vi "Parse MAVLink Message Simple.vi"(8 "error in (no error)":errorcluster, 10 "Aircraft ID":u8, 11 "Mavlink Message":string) -> (0 "error in (no error) 2":errorcluster)   [LabVIEW 2014]
uses:
  Controls/MAVLink Command ACK.ctl
  Aircraft Information/Controls/Drone Information.ctl
  Aircraft Information/Controls/Base Mode.ctl
  Aircraft Information/Controls/Aircraft Mode.ctl
  Aircraft Information/Controls/Aircraft Extra Data.ctl
  Controls/MAVLink Optical Flow.ctl
  Controls/MAVLink EKF Status Report.ctl
  Aircraft Information/Controls/Aircraft Sensor Status Data.ctl
  GUI Design/Indicators/Sensor Status LED CLuster.ctl
  GUI Design/Indicators/Status LED.ctl
  Aircraft Information/Controls/Aircraft GPS Data.ctl
  Aircraft Information/Controls/GPS Fix Type.ctl
  Aircraft Information/Controls/Aircraft Attitude Data.ctl
  Controls/MAVLink Recieved Param.ctl
  Aircraft Information/Sub VI/Set Aircraft System Status.vi
  Aircraft Information/Sub VI/Set Aircraft Information.vi
  Aircraft Information/Sub VI/Set Aircraft Extra Data.vi
  Aircraft Information/Sub VI/Set Aircraft GPS.vi
  Aircraft Information/Sub VI/Set Aircraft Attitude.vi
panel:
  out "output cluster":T1
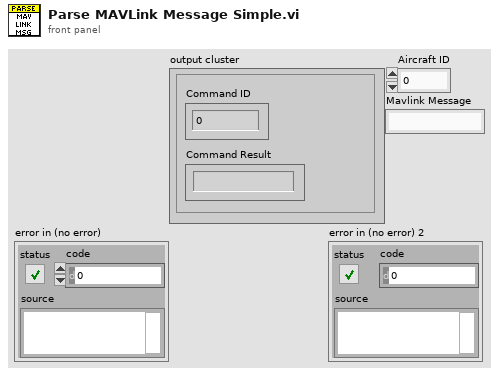
[diagram p1: front panel]
types:
  T1 = typedef "MAVLink Command ACK.ctl" = cluster{"Command ID":u16, "Command Result":string}
  T2 = typedef "Aircraft Attitude Data.ctl" = cluster{"Roll":sgl, "Pitch":sgl, "Yaw":sgl, "Timestamp":u32, "Update Frequency":dbl, "Altitude":sgl}
  T3 = typedef "Aircraft GPS Data.ctl" = cluster{"Latitude (degrees)":dbl, "Longitude (degrees)":dbl, "Altitude (m)":dbl, "Fix Type":T4, "HDOP (cm)":u16, "VDOP (cm)":u16, "Ground Speed (m/s)":dbl, "Coarse Over Ground (degrees)":u16, "Number of Satellites":u8}
  T4 = typedef "GPS Fix Type.ctl" = enum16{"No Fix 0", "No Fix 1", "2D Fix", "3D Fix", "DGPS", "RTK"}
  T5 = typedef "Aircraft Sensor Status Data.ctl" = cluster{"Sensor Status":T6, "CPU Load (%)":dbl, "Battery Voltage (V)":dbl, "Battery Current (A)":dbl, "Battery Remaining (%)":dbl, "Communication Drop Rate (%)":dbl, "Communication Errors (%)":dbl, "Status text":string}
  T6 = typedef "Sensor Status LED CLuster.ctl" = cluster{"3D Gyro":u32, "3D Accel":u32, "3D Mag":u32, "Abs. Pressure":u32, "Diff. Pressure":u32, "GPS":T7, "Optical Flow":u32, "Vision Position":u32, "Laser Position":u32, "External Ground Truth":u32, "Angular Rate Control":u32, "Attitude Stabilisation":u32, "Yaw Position":u32, "Z Altitude Control":u32, "XY Position Control":u32, "Motor Outputs":u32, "RC Receiver":u32, "3D Gyro 2":u32, "3D Accel 2":u32, "3D Mag 2":u32, "Geofence":u32, "AHRS":u32, "Terrain":u32}
  T7 = typedef "Status LED.ctl" = u32
  T8 = typedef "Aircraft Extra Data.ctl" = cluster{"Optical Flow":T9, "RNGFND Distance (m)":sgl, "RNGFND Voltage":sgl, "EKF Status Report":T10}
  T9 = typedef "MAVLink Optical Flow.ctl" = cluster{"Time (usec)":u64, "Flow Comp mx":sgl, "Flow Comp my":sgl, "Ground Distance (m)":sgl, "Flow x":i16, "Flow y":i16, "Sensord ID":u8, "Quality":u8}
  T10 = typedef "MAVLink EKF Status Report.ctl" = cluster{"EKF Status Flags":cluster{"Attitude Estimate":bool, "Horizontal Velocity":bool, "Vertical Velocity":bool, "Horizontal POS Relative":bool, "Horizontal POS Absolute":bool, "Vertical POS Relative":bool, "Vertical POS Absolute":bool, "Vertical POS AGL":bool, "Contstant POS Mode":bool, "Predicted Horizontal POS Relative":bool, "Predicted Horizontal POS Absolute":bool}, "Velocity Variance":sgl, "Horizontal POS Variance":sgl, "Vertical POS Variance":sgl, "Compass Variance":sgl, "Terrain Altitude Variance":sgl}
  T11 = typedef "Drone Information.ctl" = cluster{"Aircraft ID":u8, "Tag ID":string, "System Status":string, "Base Mode":T12, "Armed/Disarmed":bool, "Battery Voltage":dbl, "Control Mode":T13, "Initialisation":u8, "Coms with aircraft good":bool, "Mode":string, "Mission Uploaded":bool}
  T12 = typedef "Base Mode.ctl" = cluster{"Custom Mode":bool, "Test Enabled":bool, "Autonomous Mode":bool, "Guided Mode":bool, "Stabilization Enabled":bool, "HIL Enabled":bool, "Manual Mode":bool, "Arm":bool}
  T13 = typedef "Aircraft Mode.ctl" = enum16{"Loiter", "Stabalise", "Failsafe", "Emergency Stop"}
  T14 = typedef "MAVLink Recieved Param.ctl" = cluster{"Param ID":string, "Param Value":sgl, "Param Type":u8, "Param Count":u16, "Param Index":u16}
  T15 = enum16{"ALL", "RAW_SENSORS", "EXTENDED_STATUS", "RC_CHANNELS", "RAW_CONTROLLER", "POSITION", "EXTRA1", "EXTRA2", "EXTRA3"}
  T16 = cluster{"x acc":i16, "y acc":i16, "z acc":i16, "x gyro":i16, "y gyro":i16, "z gyro":i16, "x mag":i16, "y mag":i16, "z mag":i16}
  T17 = cluster{"Channel 1":u16, "Channel 2":u16, "Channel 3":u16, "Channel 4":u16, "Channel 5":u16, "Channel 6":u16, "Channel 7":u16, "Channel 8":u16}
  T18 = typedef "MAVLink Packet.ctl" = cluster{"Payload Length":u8, "Packet Sequence":u8, "System ID":u8, "Component ID":u8, "Message ID":u8, "Data":string, "Checksum":u16}
  T19 = typedef "MAVLink Heartbeat.ctl" = cluster{"custom_mode":u32, "Type":u8, "autopilot":u8, "base_mode":u8, "system_status":u8, "mavlink_version":u8, "heartbeat":bool}
  T20 = typedef "MAVLink System Status.ctl" = cluster{"onboard_control_sesnors_present":u32, "onboard_control_sesnors_enabled":u32, "onboard_control_sesnors_health":u32, "load (%*10)":u16, "voltage_battery (mV)":u16, "current_battery (mA*10)":i16, "drop_rate_comm (%*100)":u16, "error_comm":u16, "error_count1":u16, "error_count2":u16, "error_count3":u16, "error_count4":u16, "battery_remaining (%)":i8}
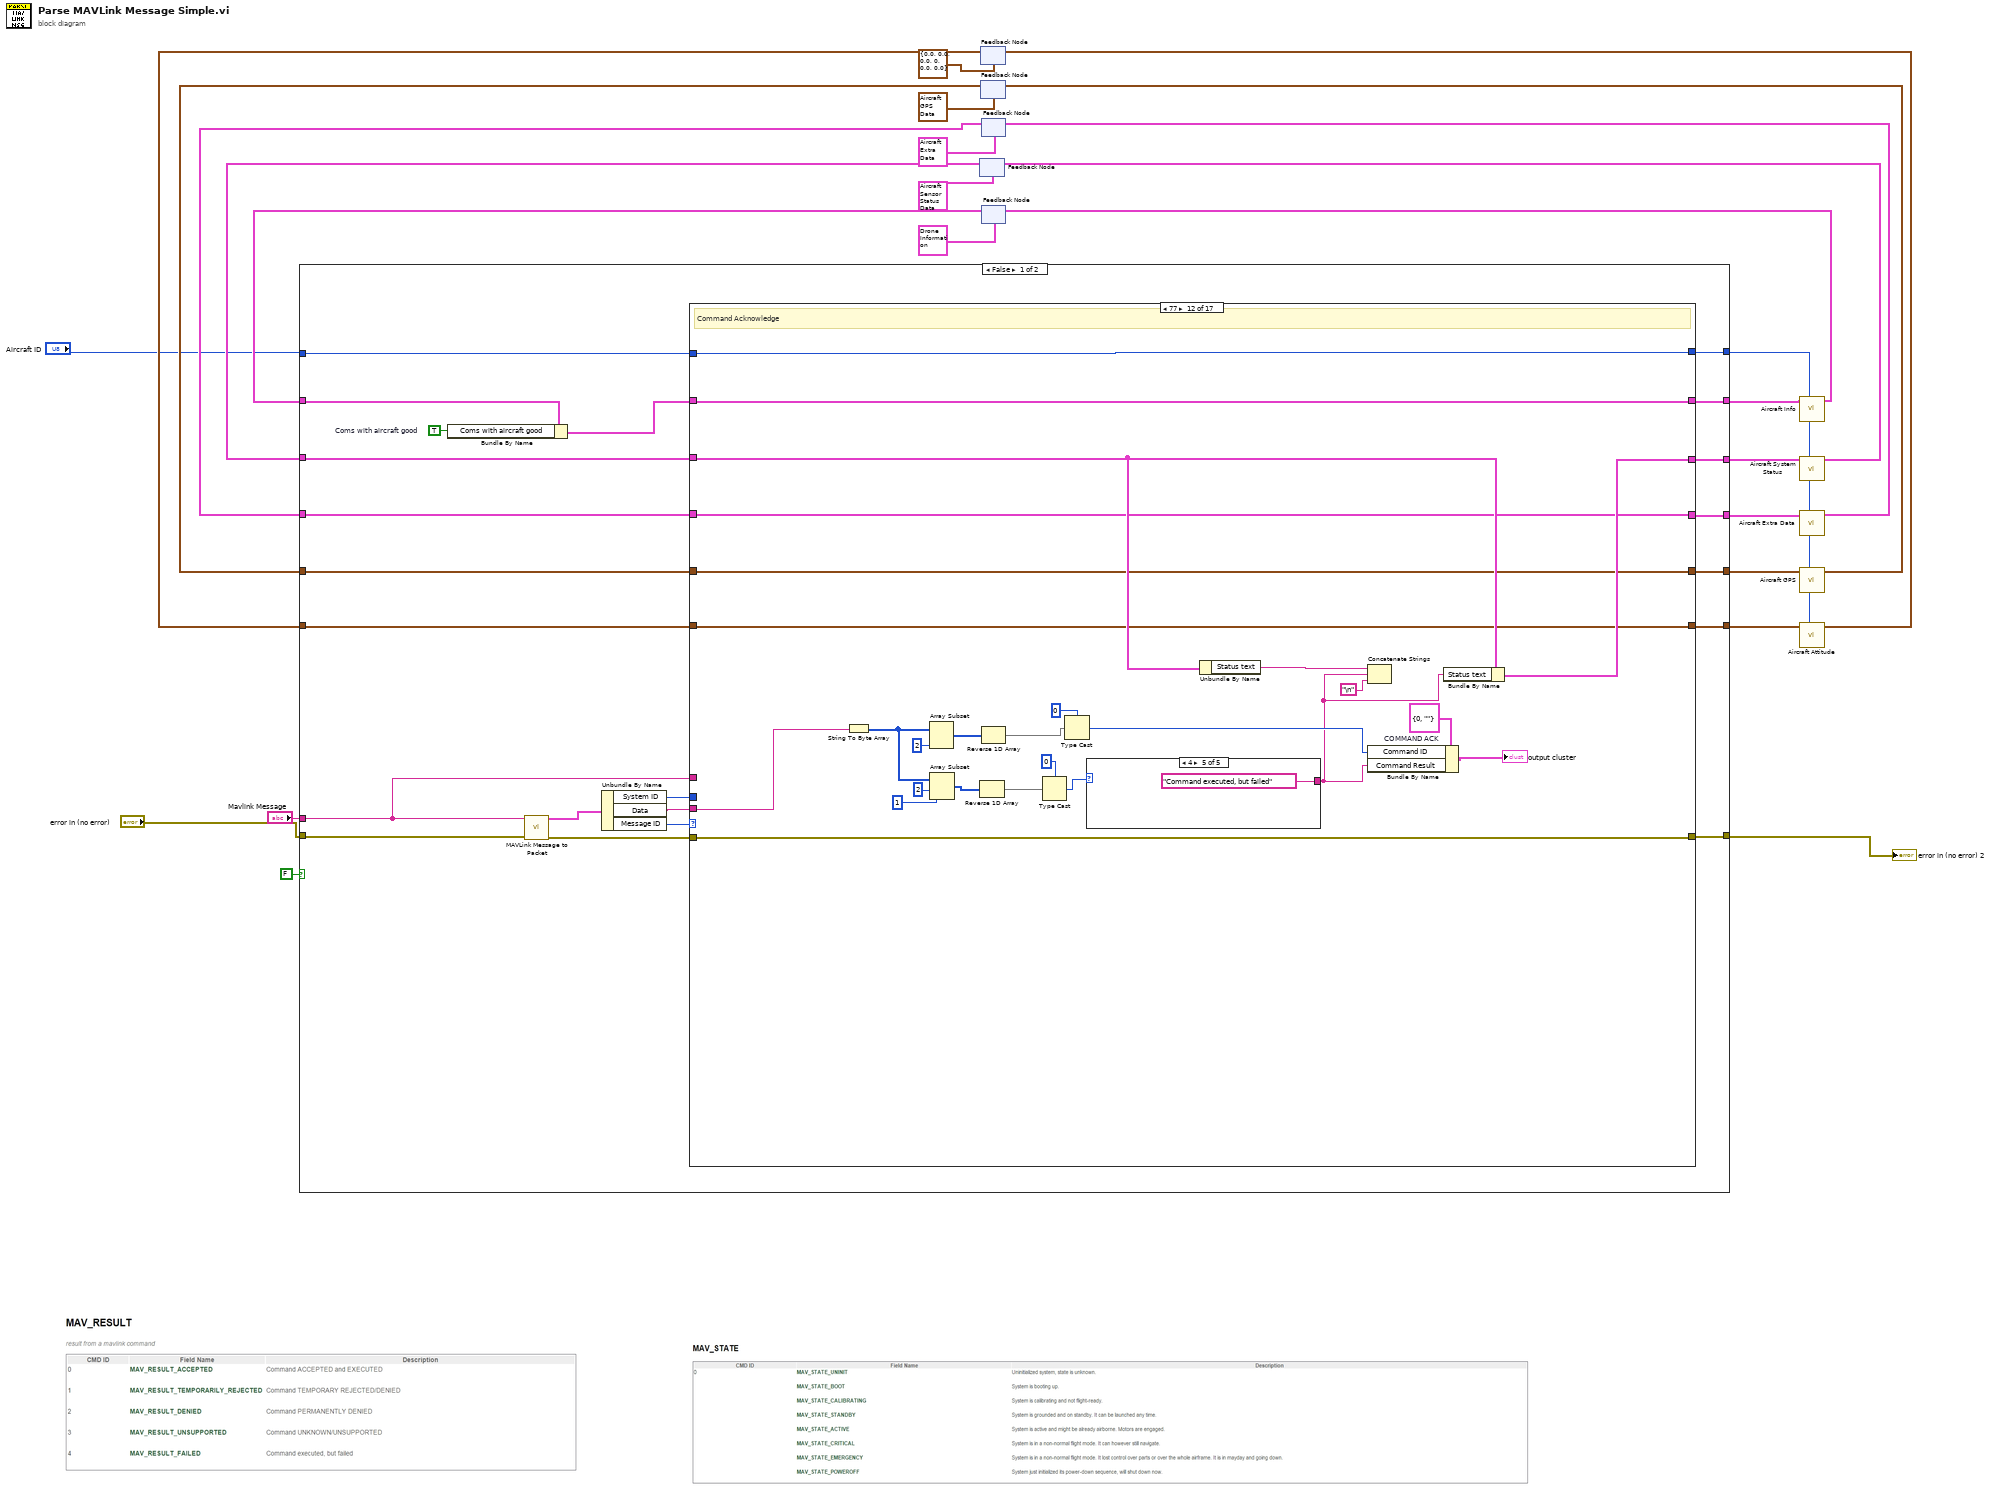
[diagram p0: block diagram]
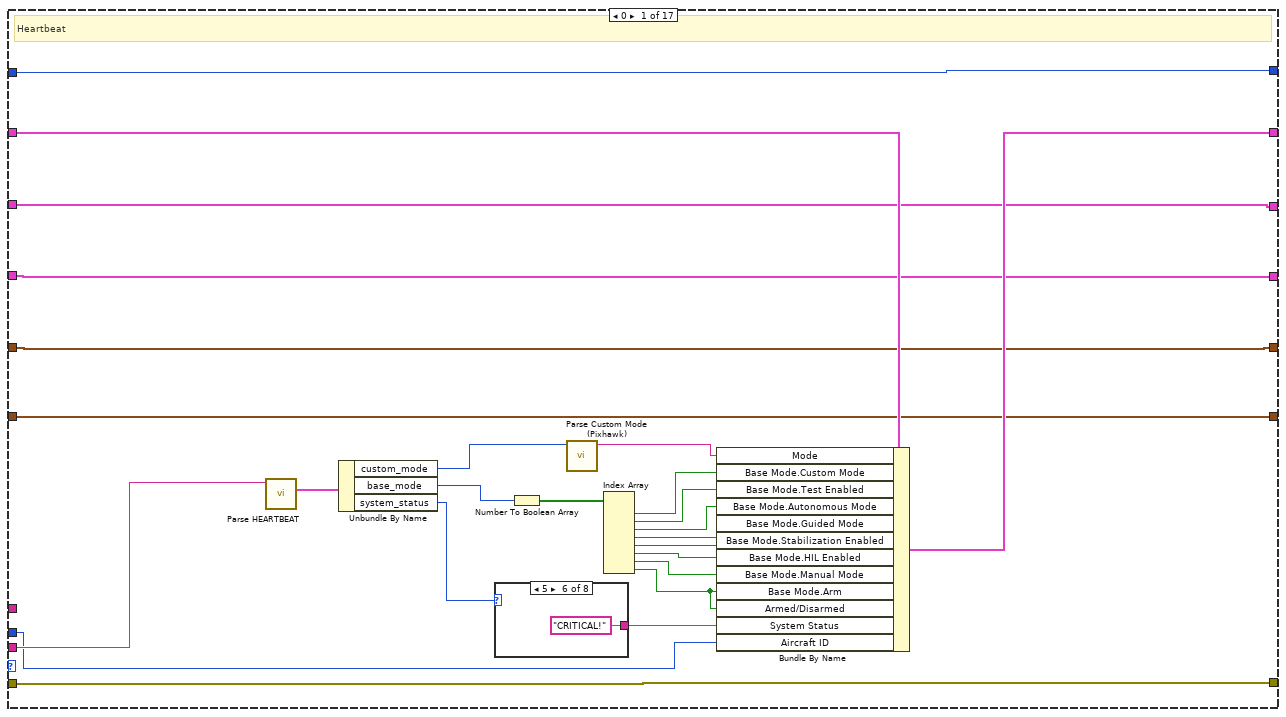
[diagram p2: hidden frame]
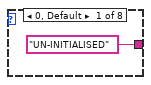
[diagram p3: hidden frame]
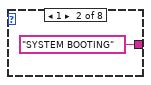
[diagram p4: hidden frame]
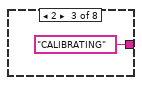
[diagram p5: hidden frame]
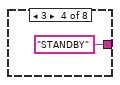
[diagram p6: hidden frame]
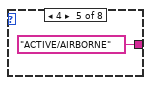
[diagram p7: hidden frame]
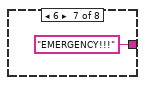
[diagram p8: hidden frame]
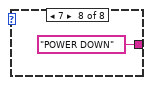
[diagram p9: hidden frame]
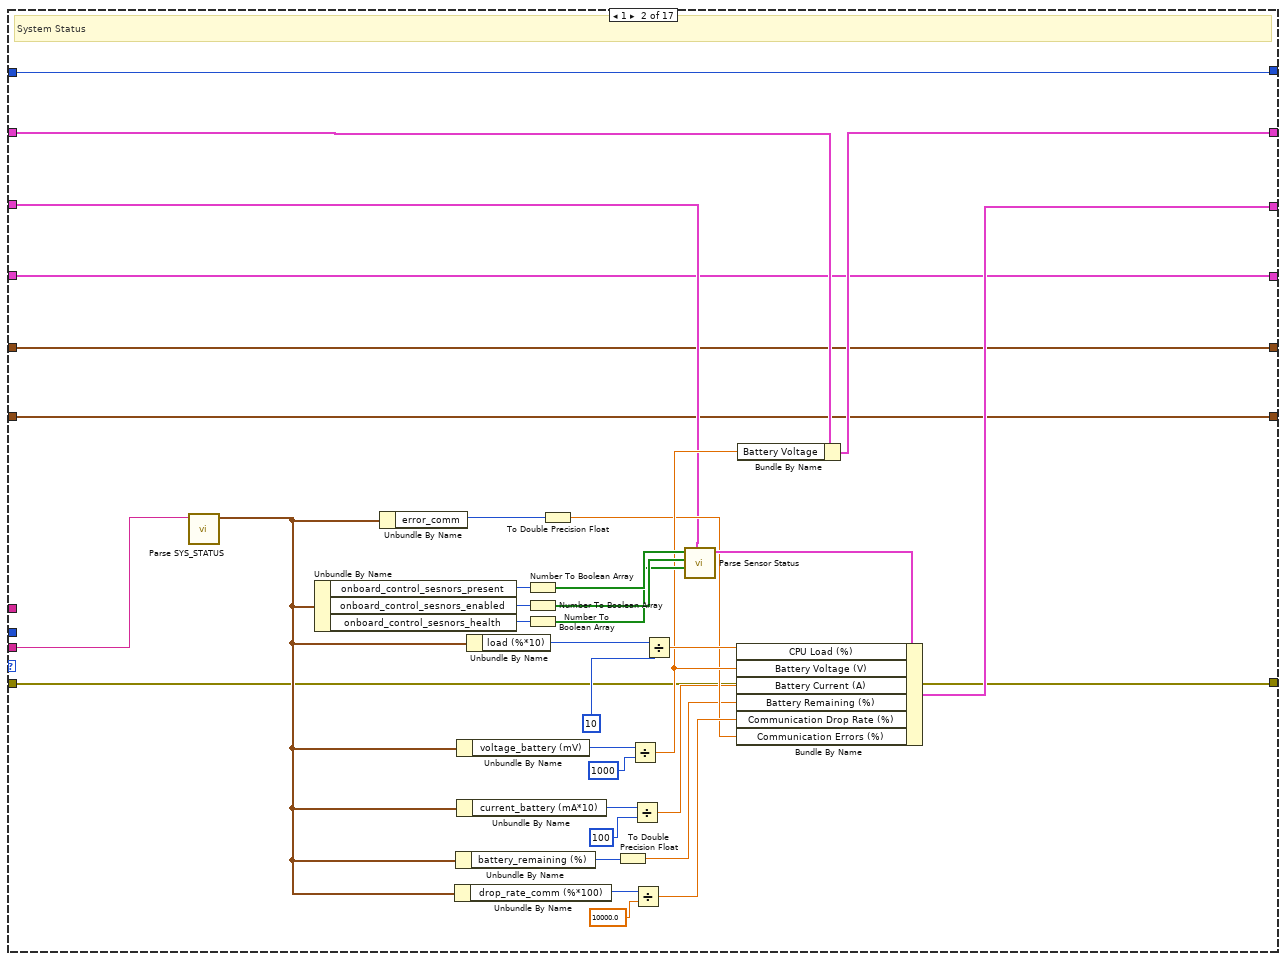
[diagram p10: hidden frame]
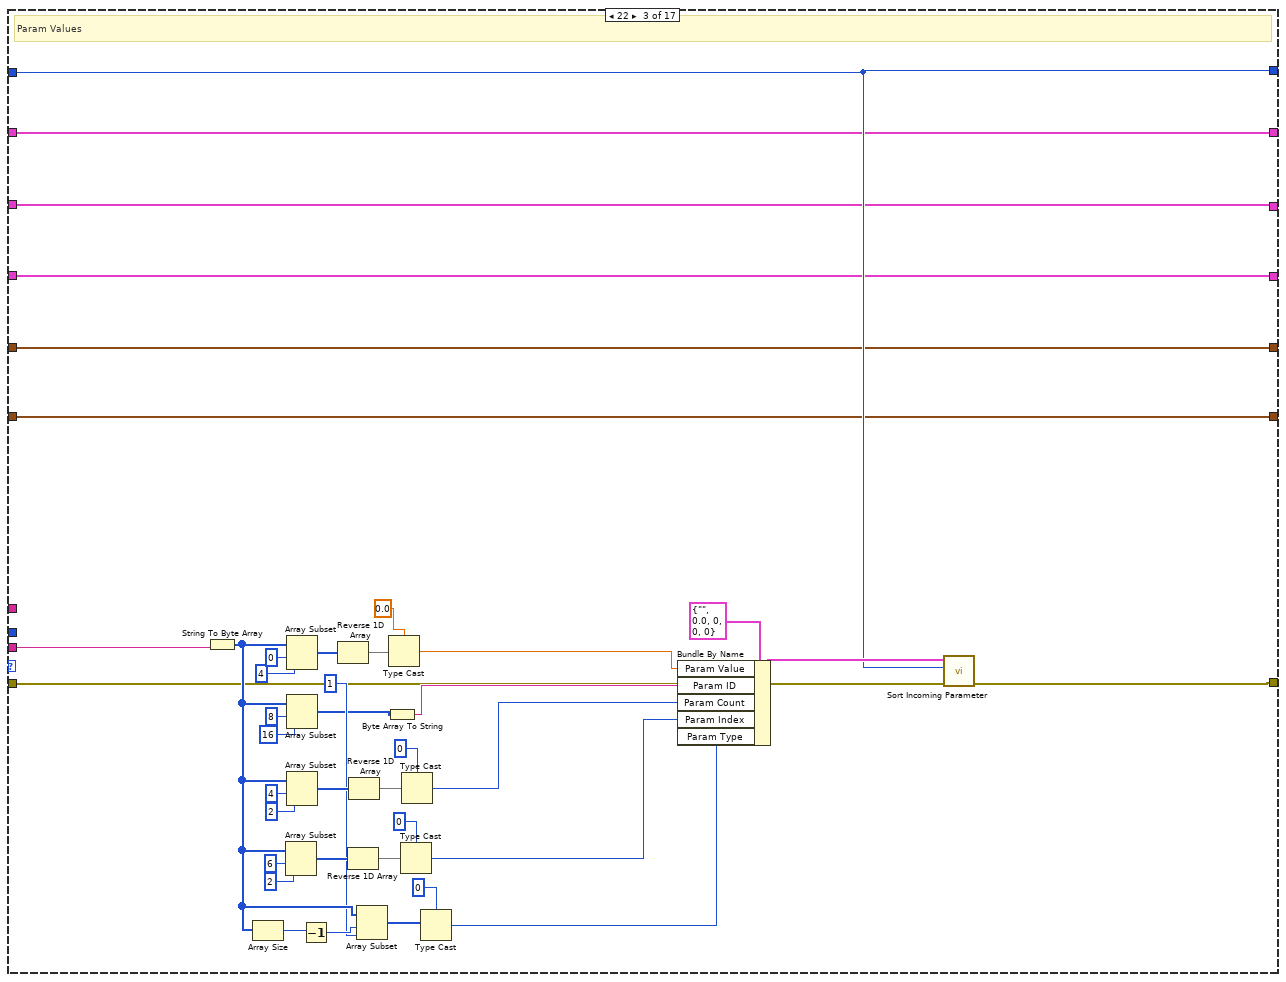
[diagram p11: hidden frame]
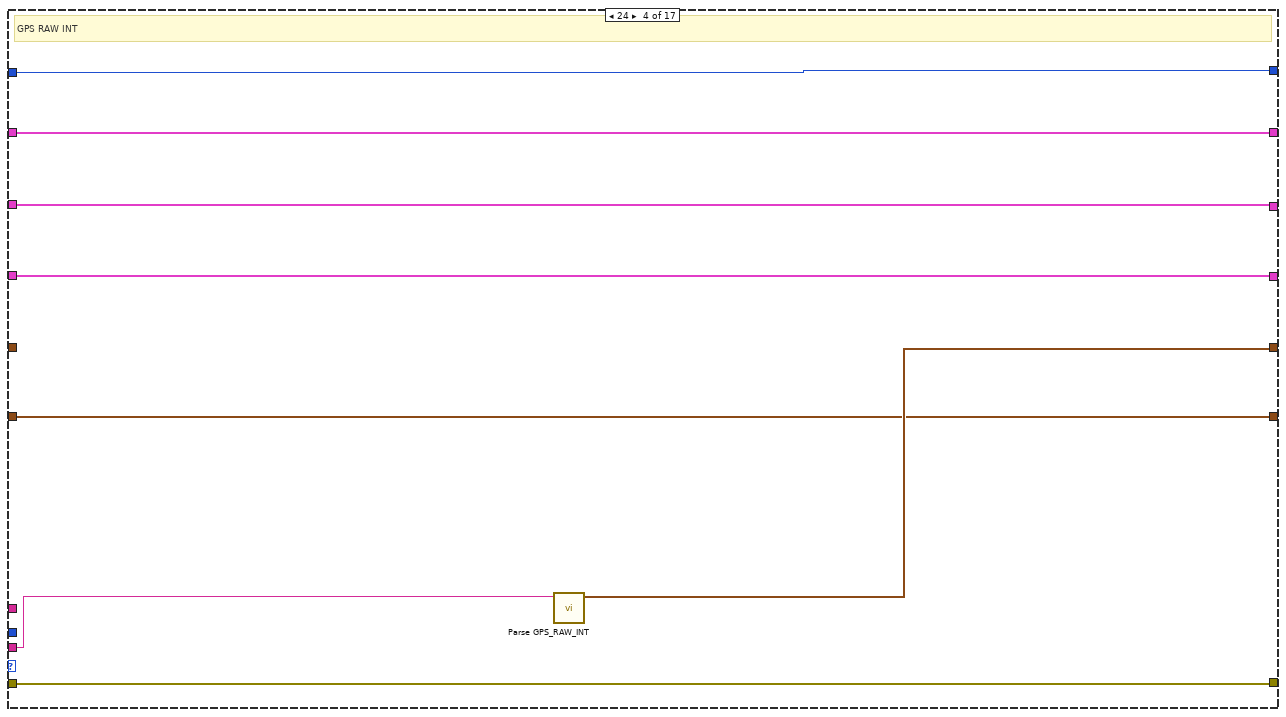
[diagram p12: hidden frame]
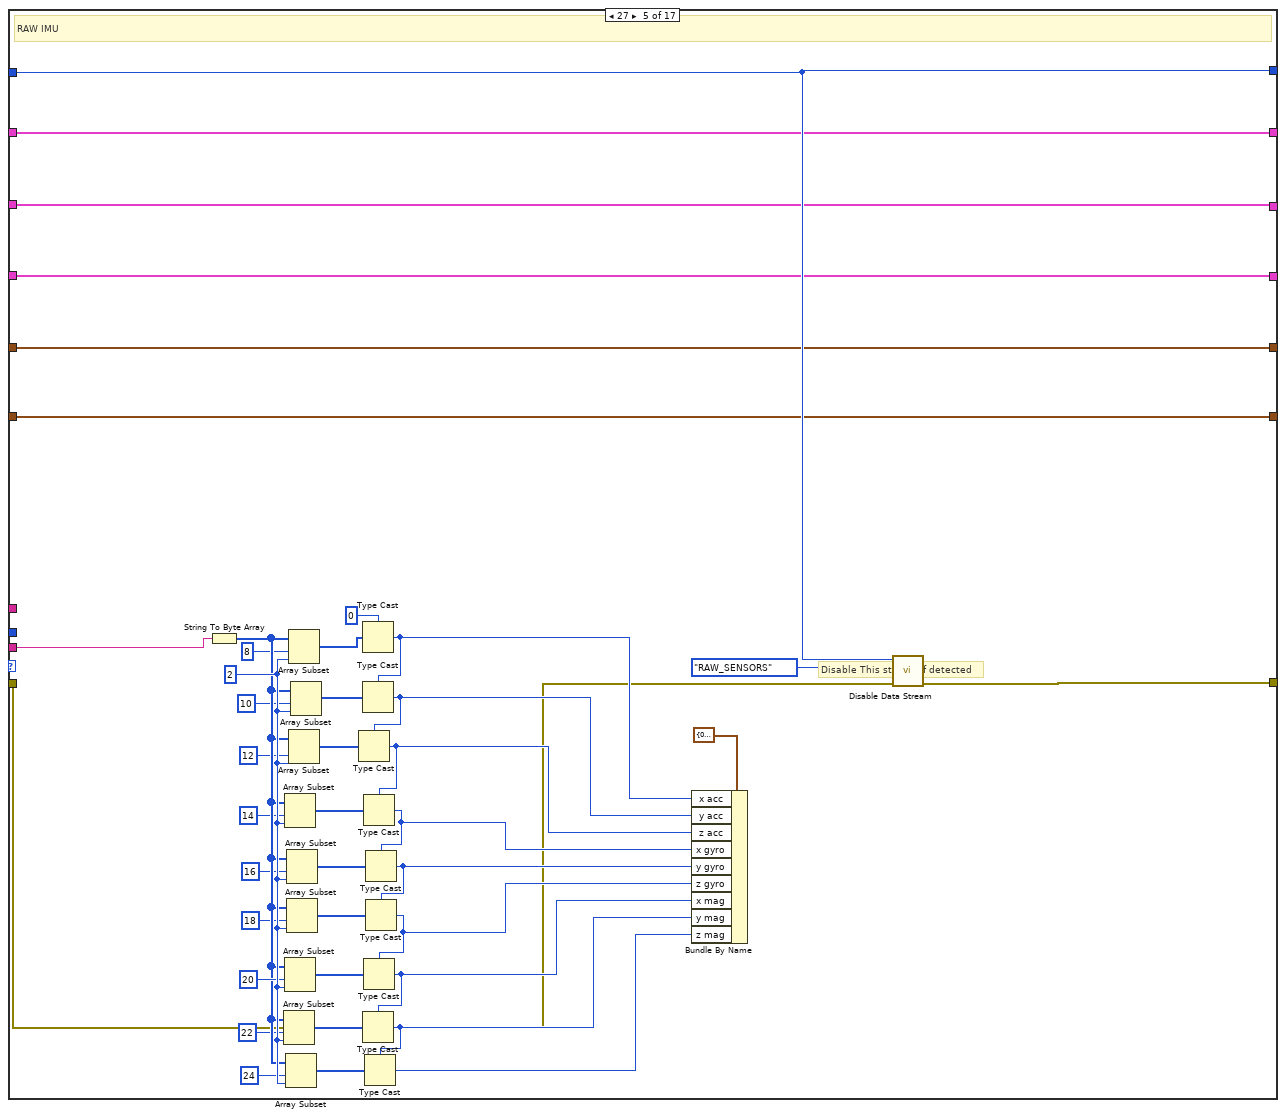
[diagram p13: hidden frame]
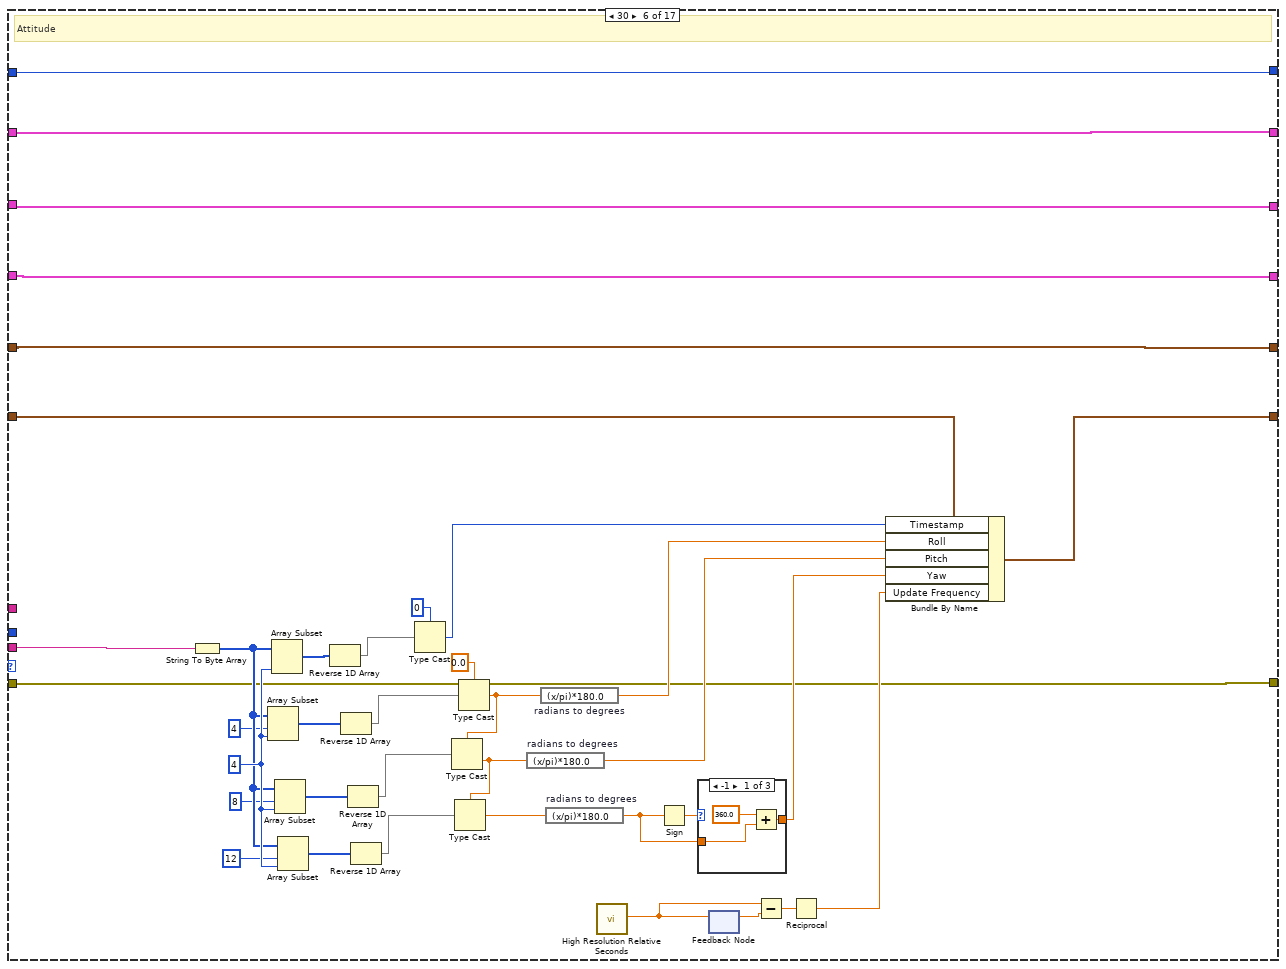
[diagram p14: hidden frame]
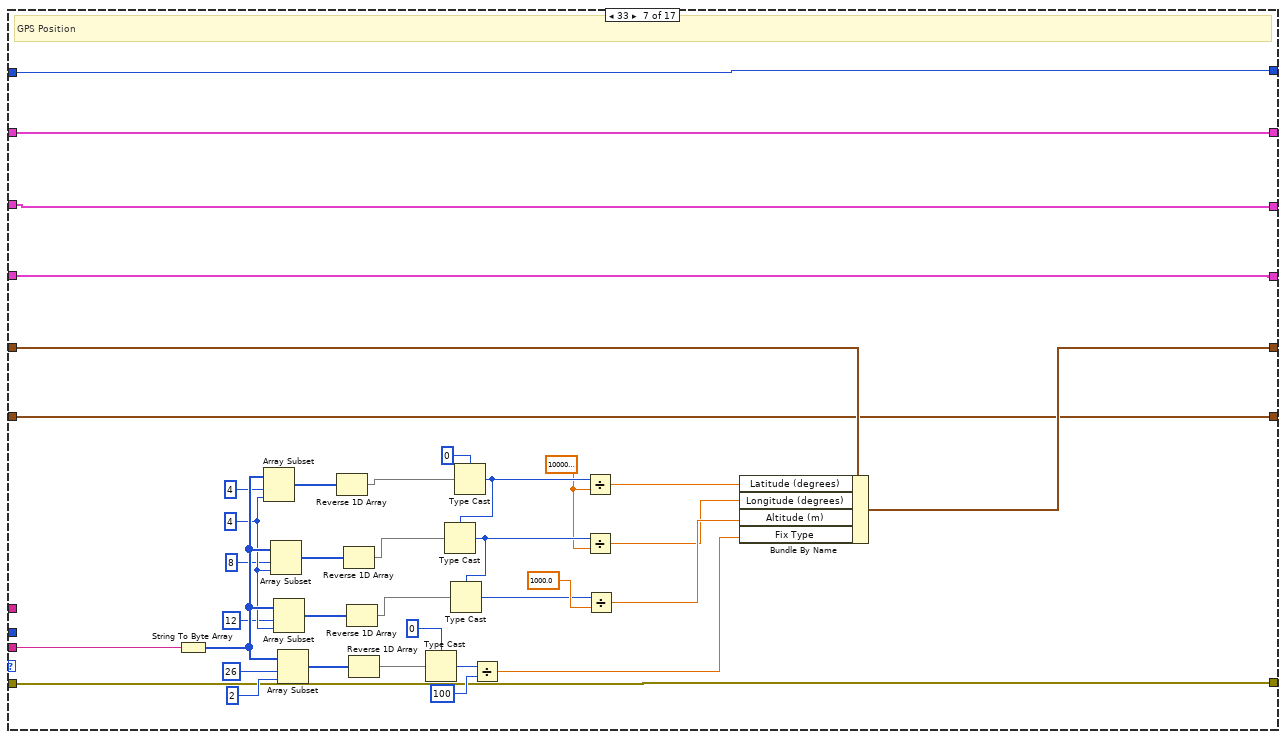
[diagram p17: hidden frame]
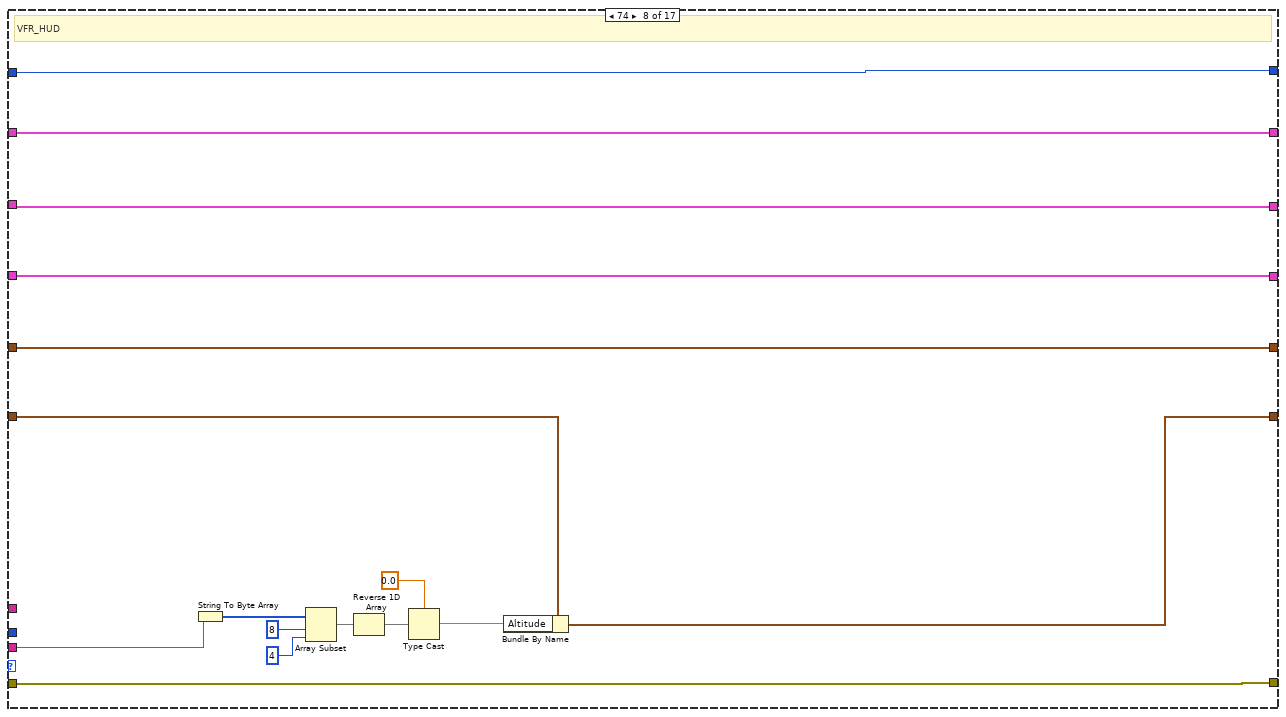
[diagram p18: hidden frame]
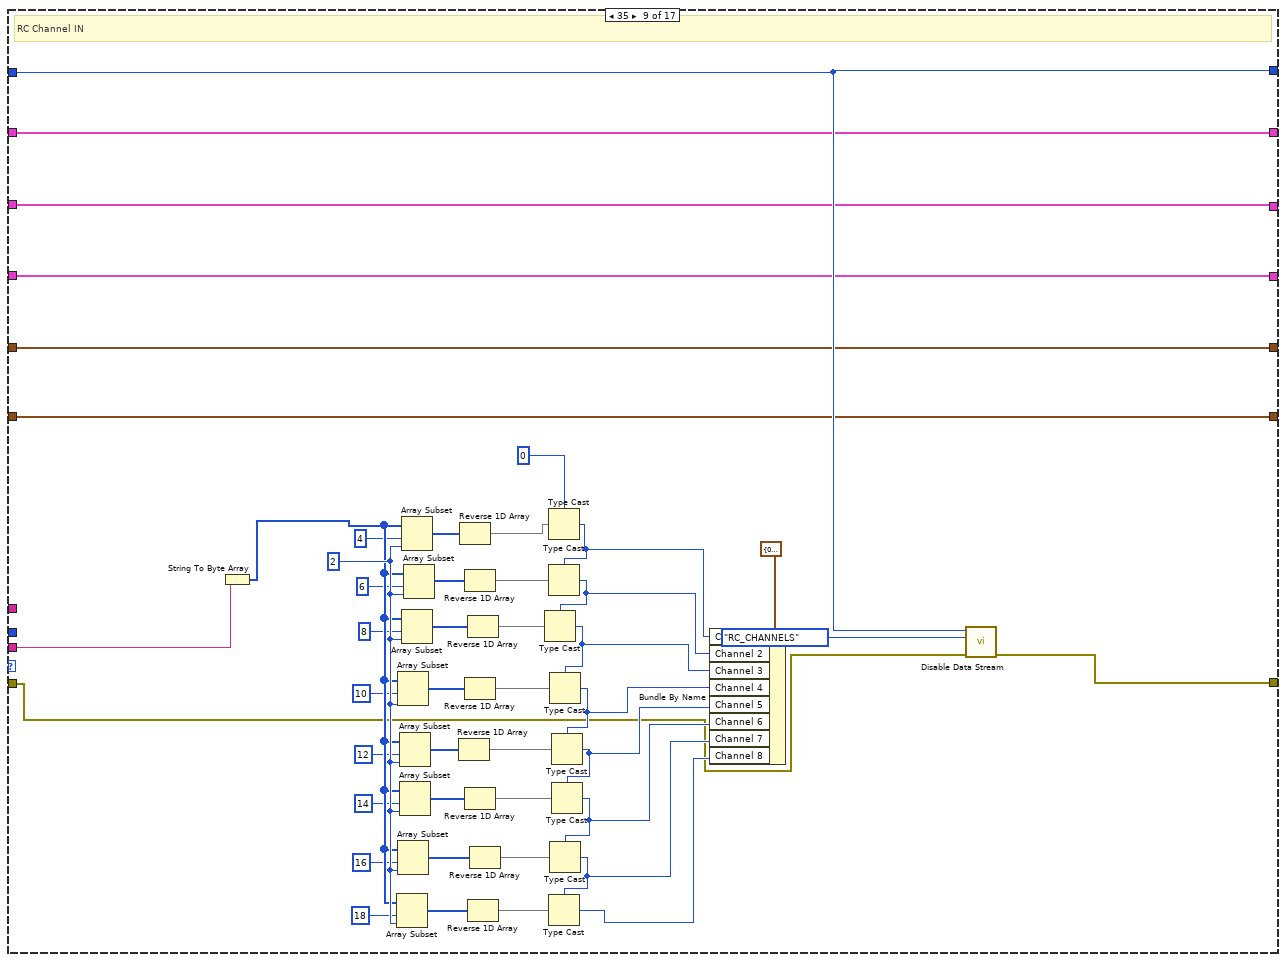
[diagram p19: hidden frame]
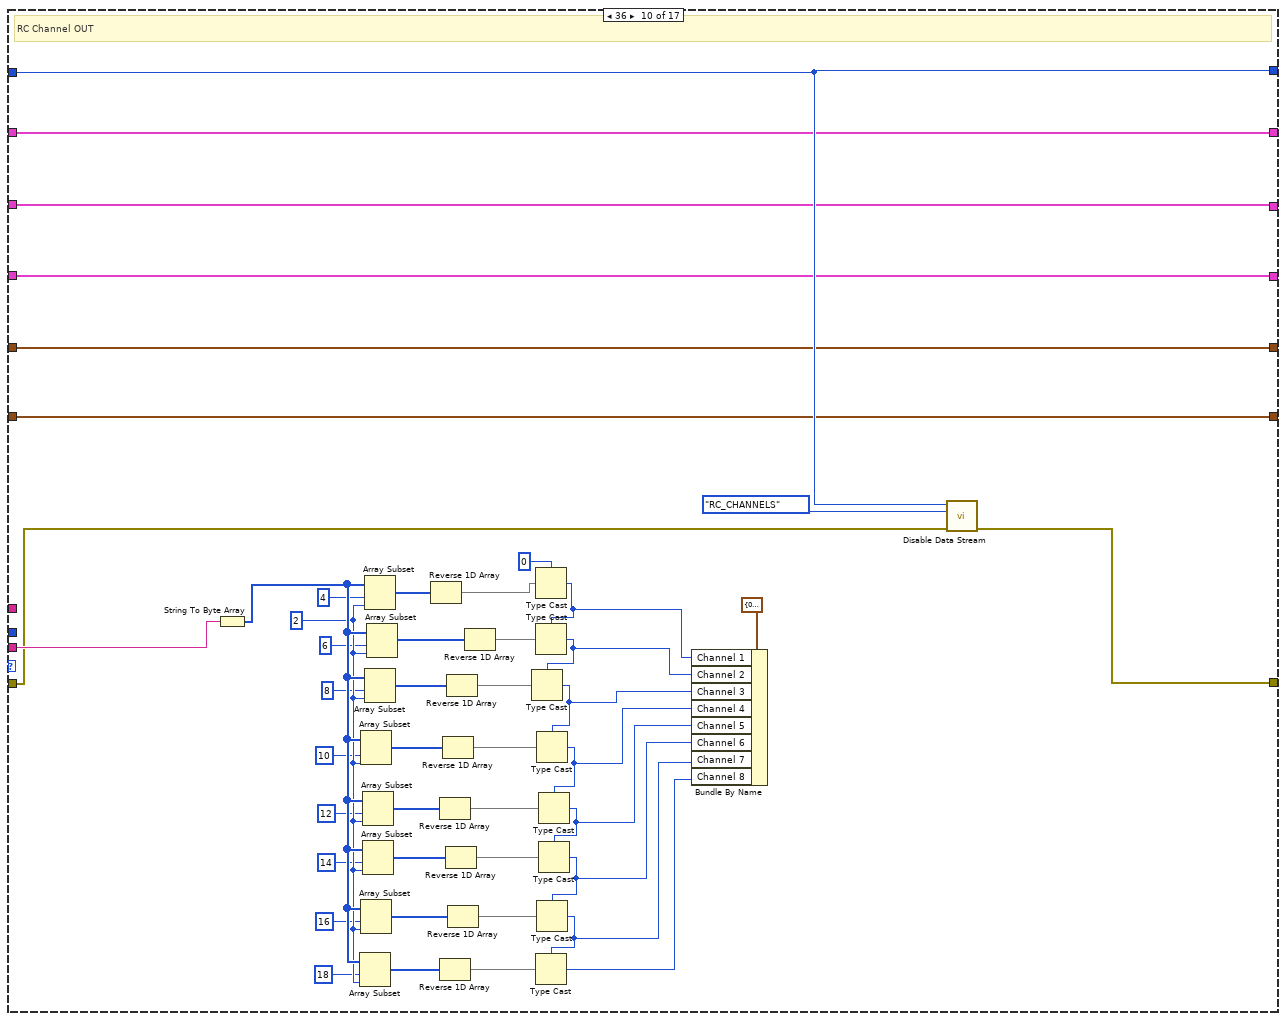
[diagram p20: hidden frame]
diagram:
  n1 = feedback #1(T5 {"Sensor Status"={"3D Gyro"=0, "3D Accel"=0, "3D Mag"=0, "Abs. Pressure"=0, "Diff. Pressure"=0, "GPS"=0, "Optical Flow"=0, "Vision Position"=0, "Laser Position"=0, "External Ground Truth"=0, "Angular Rate Control"=0, "Attitude Stabilisation"=0, "Yaw Position"=0, "Z Altitude Control"=0, "XY Position Control"=0, "Motor Outputs"=0, "RC Receiver"=0, "3D Gyro 2"=0, "3D Accel 2"=0, "3D Mag 2"=0, "Geofence"=0, "AHRS"=0, "Terrain"=0}, "CPU Load (%)"=0.0, "Battery Voltage (V)"=0.0, "Battery Current (A)"=0.0, "Battery Remaining (%)"=0.0, "Communication Drop Rate (%)"=0.0, "Communication Errors (%)"=0.0, "Status text"=""} ("System Status Out")) -> (w11:T5)
  n2 = feedback #2(T2 {"Roll"=0.0, "Pitch"=0.0, "Yaw"=0.0, "Timestamp"=0, "Update Frequency"=0.0, "Altitude"=0.0} ("Aircraft Att Data Out")) -> (w6:T2)
  n3 = feedback #3(T3 {"Latitude (degrees)"=0.0, "Longitude (degrees)"=0.0, "Altitude (m)"=0.0, "Fix Type"=enum."No Fix 0", "HDOP (cm)"=0, "VDOP (cm)"=0, "Ground Speed (m/s)"=0.0, "Coarse Over Ground (degrees)"=0, "Number of Satellites"=0} ("Aircraft Att Data Out")) -> (w7:T3)
  n4 = feedback #4(T8 {"Optical Flow"={"Time (usec)"=0, "Flow Comp mx"=0.0, "Flow Comp my"=0.0, "Ground Distance (m)"=0.0, "Flow x"=0, "Flow y"=0, "Sensord ID"=0, "Quality"=0}, "RNGFND Distance (m)"=0.0, "RNGFND Voltage"=0.0, "EKF Status Report"={"EKF Status Flags"={"Attitude Estimate"=FALSE, "Horizontal Velocity"=FALSE, "Vertical Velocity"=FALSE, "Horizontal POS Relative"=FALSE, "Horizontal POS Absolute"=FALSE, "Vertical POS Relative"=FALSE, "Vertical POS Absolute"=FALSE, "Vertical POS AGL"=FALSE, "Contstant POS Mode"=FALSE, "Predicted Horizontal POS Relative"=FALSE, "Predicted Horizontal POS Absolute"=FALSE}, "Velocity Variance"=0.0, "Horizontal POS Variance"=0.0, "Vertical POS Variance"=0.0, "Compass Variance"=0.0, "Terrain Altitude Variance"=0.0}} ("Extra Data Out")) -> (w9:T8)
  n5 = feedback #5(T11 {"Aircraft ID"=0, "Tag ID"="", "System Status"="", "Base Mode"={"Custom Mode"=FALSE, "Test Enabled"=FALSE, "Autonomous Mode"=FALSE, "Guided Mode"=FALSE, "Stabilization Enabled"=FALSE, "HIL Enabled"=FALSE, "Manual Mode"=FALSE, "Arm"=FALSE}, "Armed/Disarmed"=FALSE, "Battery Voltage"=0.0, "Control Mode"=enum."Stabalise", "Initialisation"=0, "Coms with aircraft good"=FALSE, "Mode"="", "Mission Uploaded"=FALSE} ("Aircraft Information Out")) -> (w13:T11)
  n6 = case shown="False" FALSE {
    tunnel: "error in (no error)" -> [w30 w497]
    tunnel: [w46 w497] -> w26
    tunnel: "Aircraft ID" -> [w44 w492]
    tunnel: "Mavlink Message" -> [w31 _]
    tunnel: w13 -> [w28 w491]
    tunnel: [w43 w492] -> w21
    tunnel: w11 -> [w40 w496]
    tunnel: [w41 w490] -> w25
    tunnel: [w39 w496] -> w24
    tunnel: w9 -> [w37 w495]
    tunnel: [w36 w495] -> w23
    tunnel: w7 -> [w35 w494]
    tunnel: [w34 w494] -> w22
    tunnel: w6 -> [w32 w493]
    tunnel: [w33 w493] -> w20
    frame False {
      w29 = TRUE  # Coms with aircraft good
      n7 = Bundle By Name(cluster=w28, "Coms with aircraft good"=w29) -> (w27:T11)
      n8 = call "MAVLink Message to Packet.vi"("Error In"=w30, "Message"=w31) -> ("Error Out"=w42:errorcluster, "Packet"=w45:T18)  [unwired: 8 in]
      n9 = Unbundle By Name(w45) -> ("System ID"=w38:u8, "Data"=w47:string, "Message ID"=w48:u8)
      n10 = case shown="77" w48 {
        tunnel: w47 -> [w62 w101 w155 w163 w174 w218 w255 w296 w309 w364 _ w421 w439 w450 w460 w481 _]
        tunnel: w38 -> [w53 _ _ _ _ _ _ _ _ _ _ _ _ _ _ _ _]
        tunnel: w42 -> [w54 w82 w123 w157 w171 w206 w254 w287 w307 w352 w392 w404 w434 w444 w456 w463 w488]
        tunnel: [w54 w82 w119 w157 w172 w206 w254 w287 w308 w353 w392 w404 w434 w444 w456 w463 w488] -> w46
        tunnel: w27 -> [w63 w102 w121 w161 w167 w205 w250 w286 w303 w349 w396 w406 w432 w443 w454 w464 w486]
        tunnel: w44 -> [w58 w89 w122 w162 w169 w212 w253 w291 w305 w351 w398 w408 w437 w447 w458 w468 w487]
        tunnel: w31 -> [_ _ _ _ _ _ _ _ _ _ _ _ _ _ _ _ _]
        tunnel: [w58 w89 w122 w162 w169 w212 w253 w291 w305 w351 w398 w408 w437 w447 w458 w468 w487] -> w43
        tunnel: [w55 w88 w121 w161 w167 w205 w250 w286 w303 w349 w396 w406 w432 w443 w454 w464 w486] -> w41
        tunnel: w40 -> [w52 w87 w120 w160 w166 w208 w249 w285 w302 w348 w395 w407 w431 w442 w453 w467 w485]
        tunnel: [w52 w86 w120 w160 w166 w208 w249 w285 w302 w348 w395 w405 w431 w442 w453 w466 w485] -> w39
        tunnel: w37 -> [w51 w85 w118 w159 w165 w207 w248 w284 w301 w347 w394 w401 w436 w446 w457 w465 w484]
        tunnel: [w51 w85 w118 w159 w165 w207 w248 w284 w301 w347 w394 w401 w435 w445 w455 w465 w484] -> w36
        tunnel: w35 -> [w50 w84 w117 _ w168 w211 w252 w290 w304 w350 w397 w402 w433 w441 w452 w462 w483]
        tunnel: [w50 w84 w117 w158 w168 w211 w251 w290 w304 w350 w397 w402 w433 w441 w452 w462 w483] -> w34
        tunnel: [w49 w83 w116 w156 w164 w209 w247 w288 w300 w346 w393 w400 w430 w440 w451 w461 w482] -> w33
        tunnel: w32 -> [w49 w83 w116 w156 w164 w210 w247 w289 w300 w346 w393 w400 w430 w440 w451 w461 w482]
        frame 0 {
          # "Heartbeat"
          n11 = call "Parse HEARTBEAT.vi"("Data"=w62) -> ("Heartbeat"=w61:T19)  [unwired: 10 in]
          n12 = Unbundle By Name(w61) -> ("custom_mode"=w57:u32, "base_mode"=w59:u8, "system_status"=w60:u8)
          n13 = case shown="5" w60 {
            tunnel: ["UN-INITIALISED" "SYSTEM BOOTING" "CALIBRATING" "STANDBY" "ACTIVE/AIRBORNE" "CRITICAL!" "EMERGENCY!!!" "POWER DOWN"] -> w64
            frame 0, Default {
            }
            frame 1 {
            }
            frame 2 {
            }
            frame 3 {
            }
            frame 4 {
            }
            frame 5 {
            }
            frame 6 {
            }
            frame 7 {
            }
          }
          n14 = Number To Boolean Array(number=w59) -> (Boolean array=w73:bool[])
          n15 = call "Parse Custom Mode (Pixhawk).vi"("custom mode"=w57) -> ("Custom Mode"=w56:string)  [unwired: 9 in, 1 out]
          n16 = Index Array(array=w73) -> (element #1=w72:bool, element #2=w71:bool, element #3=w70:bool, element #4=w69:bool, element #5=w68:bool, element #6=w67:bool, element #7=w66:bool, element #8=w65:bool)  [unwired: 8 in]
          n17 = Bundle By Name(cluster=w63, "Mode"=w56, "Base Mode.Custom Mode"=w72, "Base Mode.Test Enabled"=w71, "Base Mode.Autonomous Mode"=w70, "Base Mode.Guided Mode"=w69, "Base Mode.Stabilization Enabled"=w68, "Base Mode.HIL Enabled"=w67, "Base Mode.Manual Mode"=w66, "Base Mode.Arm"=w65, "Armed/Disarmed"=w65, "System Status"=w64, "Aircraft ID"=w53) -> (w55:T11)
        }
        frame 1 {
          # "System Status"
          n18 = call "Parse SYS_STATUS.vi"("Data"=w101) -> ("System Status"=w91:T20)  [unwired: 10 in]
          n19 = Unbundle By Name(w91) -> ("onboard_control_sesnors_present"=w100:u32, "onboard_control_sesnors_enabled"=w99:u32, "onboard_control_sesnors_health"=w98:u32)
          n20 = Unbundle By Name(w91) -> ("error_comm"=w90:u16)
          n21 = Unbundle By Name(w91) -> ("drop_rate_comm (%*100)"=w92:u16)
          n22 = Unbundle By Name(w91) -> ("battery_remaining (%)"=w94:i8)
          n23 = Unbundle By Name(w91) -> ("voltage_battery (mV)"=w96:u16)
          n24 = Unbundle By Name(w91) -> ("current_battery (mA*10)"=w95:i16)
          n25 = Unbundle By Name(w91) -> ("load (%*10)"=w97:u16)
          n26 = Number To Boolean Array(number=w100) -> (Boolean array=w113:bool[])
          n27 = Number To Boolean Array(number=w99) -> (Boolean array=w112:bool[])
          n28 = Number To Boolean Array(number=w98) -> (Boolean array=w111:bool[])
          n29 = To Double Precision Float(number=w90) -> (double precision float=w104:dbl)
          n30 = To Double Precision Float(number=w94) -> (double precision float=w93:dbl)
          n31 = Divide(x=w96, y=u16 1000) -> (x/y=w107:dbl)
          n32 = Divide(x=w95, y=i16 100) -> (x/y=w103:dbl)
          n33 = Divide(x=w92, y=10000.0) -> (x/y=w105:dbl)
          n34 = Divide(x=w97, y=u16 10) -> (x/y=w108:dbl)
          n35 = call "Parse Sensor Status.vi"("Aircraft System Status"=w87, "Healthy"=w111, "Enabled"=w112, "Present"=w113) -> ("Aircraft System Status Out"=w110:T5)  [unwired: 7 in]
          n36 = Bundle By Name(cluster=w110, "CPU Load (%)"=w108, "Battery Voltage (V)"=w107, "Battery Current (A)"=w103, "Battery Remaining (%)"=w93, "Communication Drop Rate (%)"=w105, "Communication Errors (%)"=w104) -> (w86:T5)
          n37 = Bundle By Name(cluster=w102, "Battery Voltage"=w107) -> (w88:T11)
        }
        frame 22 {
          # "Param Values"
          n38 = String To Byte Array(string=w155) -> (unsigned byte array=w134:u8[])
          n39 = Array Size(array=w134) -> (size(s)=w135:i32)
          n40 = Array Subset(array=w134, index=6, length=2) -> (w140:u8[])
          n41 = Array Subset(array=w134, index=0, length=4) -> (w152:u8[])
          n42 = Array Subset(array=w134, index=8, length=16) -> (w126:u8[])
          n43 = Array Subset(array=w134, index=4, length=2) -> (w145:u8[])
          n44 = Decrement(x=w135) -> (x-1=w133:i32)
          n45 = Reverse 1D Array(array=w152) -> (reversed array=w151:u8[])
          n46 = Reverse 1D Array(array=w140) -> (reversed array=w141:u8[])
          n47 = Reverse 1D Array(array=w145) -> (reversed array=w144:u8[])
          n48 = Array Subset(array=w134, index=w133, length=1) -> (w131:u8[])
          n49 = Byte Array To String(unsigned byte array=w126) -> (string=w128:string)
          n50 = Type Cast(type=sgl 0.0, x=w151) -> (*(type *) &x=w127:sgl)
          n51 = Type Cast(type=u16 0, x=w141) -> (*(type *) &x=w136:u16)
          n52 = Type Cast(type=u16 0, x=w144) -> (*(type *) &x=w142:u16)
          n53 = Type Cast(type=u8 0, x=w131) -> (*(type *) &x=w129:u8)
          n54 = Bundle By Name(cluster=T14 {"Param ID"="", "Param Value"=0.0, "Param Type"=0, "Param Count"=0, "Param Index"=0} ("Param Value Out"), "Param Value"=w127, "Param ID"=w128, "Param Count"=w142, "Param Index"=w136, "Param Type"=w129) -> (w125:T14)
          n55 = call "Sort Incoming Parameter.vi"("Error In"=w123, "Aircraft ID"=w122, "Param Value"=w125) -> ("Error Out"=w119:errorcluster)  [unwired: 8 in]
        }
        frame 24 {
          # "GPS RAW INT"
          n56 = call "Parse GPS_RAW_INT.vi"("Data"=w163) -> ("GPS Data Out"=w158:T3)  [unwired: 10 in]
        }
        frame 27 {
          w195 = 2 ("length")
          # "Disable This stream if detected"
          # "RAW IMU"
          n57 = String To Byte Array(string=w174) -> (unsigned byte array=w193:u8[])
          n58 = Array Subset(array=w193, index=22, length=w195) -> (w188:u8[])
          n59 = Array Subset(array=w193, index=14, length=w195) -> (w177:u8[])
          n60 = Array Subset(array=w193, index=20, length=w195) -> (w192:u8[])
          n61 = Array Subset(array=w193, index=24, length=w195) -> (w191:u8[])
          n62 = Array Subset(array=w193, index=16, length=w195) -> (w184:u8[])
          n63 = Array Subset(array=w193, index=18, length=w195) -> (w187:u8[])
          n64 = Array Subset(array=w193, index=8, length=w195) -> (w182:u8[])
          n65 = Array Subset(array=w193, index=12, length=w195) -> (w176:u8[])
          n66 = Array Subset(array=w193, index=10, length=w195) -> (w183:u8[])
          n67 = Type Cast(type=i16 0, x=w182) -> (*(type *) &x=w196:i16)
          n68 = Type Cast(type=w196, x=w183) -> (*(type *) &x=w197:i16)
          n69 = Type Cast(type=w197, x=w176) -> (*(type *) &x=w198:i16)
          n70 = Type Cast(type=w198, x=w177) -> (*(type *) &x=w204:i16)
          n71 = Type Cast(type=w204, x=w184) -> (*(type *) &x=w199:i16)
          n72 = Type Cast(type=w199, x=w187) -> (*(type *) &x=w200:i16)
          n73 = Type Cast(type=w200, x=w192) -> (*(type *) &x=w201:i16)
          n74 = Type Cast(type=w201, x=w188) -> (*(type *) &x=w202:i16)
          n75 = Type Cast(type=w202, x=w191) -> (*(type *) &x=w203:i16)
          n76 = Bundle By Name(cluster=T16 {"x acc"=0, "y acc"=0, "z acc"=0, "x gyro"=0, "y gyro"=0, "z gyro"=0, "x mag"=0, "y mag"=0, "z mag"=0} ("Raw IMU"), "x acc"=w196, "y acc"=w197, "z acc"=w198, "x gyro"=w204, "y gyro"=w199, "z gyro"=w200, "x mag"=w201, "y mag"=w202, "z mag"=w203) -> ()  [unwired: 1 out]
          n77 = call "Disable Data Stream.vi"("error in (no error)"=w171, "req_stream_id"=T15."RAW_SENSORS", "Aircraft ID"=w169) -> ("error out"=w172:errorcluster)  [unwired: 8 in]
        }
        frame 30 {
          w231 = 4 ("length")
          # "Attitude"
          n78 = String To Byte Array(string=w218) -> (unsigned byte array=w230:u8[])
          n79 = Array Subset(array=w230, index=4, length=w231) -> (w221:u8[])
          n80 = Array Subset(array=w230, length=w231) -> (w232:u8[])  [unwired: 1 in]
          n81 = Array Subset(array=w230, index=8, length=w231) -> (w223:u8[])
          n82 = Array Subset(array=w230, index=12, length=w231) -> (w226:u8[])
          n83 = Reverse 1D Array(array=w232) -> (reversed array=w233:u8[])
          n84 = Reverse 1D Array(array=w221) -> (reversed array=w222:u8[])
          n85 = Reverse 1D Array(array=w223) -> (reversed array=w227:u8[])
          n86 = Reverse 1D Array(array=w226) -> (reversed array=w228:u8[])
          n87 = Type Cast(type=u32 0 ("single precision float"), x=w233) -> (*(type *) &x=w217:u32)
          n88 = Type Cast(type=sgl 0.0 ("single precision float"), x=w222) -> (*(type *) &x=w235:sgl)
          n89 = Type Cast(type=w235, x=w227) -> (*(type *) &x=w236:sgl)
          n90 = Type Cast(type=w236, x=w228) -> (*(type *) &x=w237:sgl)
          n91 = expression code="(x/pi)*180.0" "radians to degrees"(w236) -> (w241:sgl)
          n92 = expression code="(x/pi)*180.0" "radians to degrees"(w235) -> (w240:sgl)
          n93 = expression code="(x/pi)*180.0" "radians to degrees"(w237) -> (w238:sgl)
          n94 = call <vilib>:"High Resolution Relative Seconds.vi"() -> ("relative seconds"=w215:dbl)
          n95 = Sign(1:w238) -> (0:w229:sgl)
          n96 = case shown="-1" w229 {
            tunnel: w238 -> [w243 w245 w246]
            tunnel: [w242 w245 w246] -> w239
            frame -1 {
              n97 = Add(x=sgl 360.0, y=w243) -> (x+y=w242:sgl)
            }
            frame 0, Default {
            }
            frame 1 {
            }
          }
          n98 = feedback-in #6(w215) -> ()
          n99 = feedback #6() -> (w216:dbl)  [unwired: 1 in]
          n100 = Subtract(x=w215, y=w216) -> (x-y=w214:dbl)
          n101 = Reciprocal(x=w214) -> (1/x=w213:dbl)
          n102 = Bundle By Name(cluster=w210, "Timestamp"=w217, "Roll"=w240, "Pitch"=w241, "Yaw"=w239, "Update Frequency"=w213) -> (w209:T2)
        }
        frame 33 {
          w266 = sgl 10000000.0
          w265 = 4 ("length")
          # "GPS Position"
          n103 = String To Byte Array(string=w255) -> (unsigned byte array=w271:u8[])
          n104 = Array Subset(array=w271, index=4, length=w265) -> (w257:u8[])
          n105 = Array Subset(array=w271, index=8, length=w265) -> (w259:u8[])
          n106 = Array Subset(array=w271, index=12, length=w265) -> (w262:u8[])
          n107 = Array Subset(array=w271, index=26, length=2) -> (w276:u8[])
          n108 = Reverse 1D Array(array=w257) -> (reversed array=w258:u8[])
          n109 = Reverse 1D Array(array=w259) -> (reversed array=w263:u8[])
          n110 = Reverse 1D Array(array=w262) -> (reversed array=w264:u8[])
          n111 = Reverse 1D Array(array=w276) -> (reversed array=w277:u8[])
          n112 = Type Cast(type=u16 0, x=w277) -> (*(type *) &x=w274:u16)
          n113 = Type Cast(type=0, x=w258) -> (*(type *) &x=w267:i32)
          n114 = Type Cast(type=w267, x=w263) -> (*(type *) &x=w268:i32)
          n115 = Type Cast(type=w268, x=w264) -> (*(type *) &x=w269:i32)
          n116 = Divide(x=w274, y=u16 100) -> (x/y=w283:dbl)
          n117 = Divide(x=w267, y=w266) -> (x/y=w280:sgl)
          n118 = Divide(x=w268, y=w266) -> (x/y=w281:sgl)
          n119 = Divide(x=w269, y=sgl 1000.0) -> (x/y=w282:sgl)
          n120 = Bundle By Name(cluster=w252, "Latitude (degrees)"=w280, "Longitude (degrees)"=w281, "Altitude (m)"=w282, "Fix Type"=w283) -> (w251:T3)
        }
        frame 74 {
          # "VFR_HUD"
          n121 = String To Byte Array(string=w296) -> (unsigned byte array=w295:u8[])
          n122 = Array Subset(array=w295, index=8, length=4) -> (w298:u8[])
          n123 = Reverse 1D Array(array=w298) -> (reversed array=w299:u8[])
          n124 = Type Cast(type=sgl 0.0 ("single precision float"), x=w299) -> (*(type *) &x=w293:sgl)
          n125 = Bundle By Name(cluster=w289, "Altitude"=w293) -> (w288:T2)
        }
        frame 35 {
          w328 = 2 ("index")
          # "RC Channel IN"
          n126 = String To Byte Array(string=w309) -> (unsigned byte array=w327:u8[])
          n127 = Array Subset(array=w327, index=18, length=w328) -> (w323:u8[])
          n128 = Array Subset(array=w327, index=10, length=w328) -> (w312:u8[])
          n129 = Array Subset(array=w327, index=16, length=w328) -> (w325:u8[])
          n130 = Array Subset(array=w327, index=12, length=w328) -> (w319:u8[])
          n131 = Array Subset(array=w327, index=14, length=w328) -> (w322:u8[])
          n132 = Array Subset(array=w327, index=4, length=w328) -> (w317:u8[])
          n133 = Array Subset(array=w327, index=8, length=w328) -> (w311:u8[])
          n134 = Array Subset(array=w327, index=6, length=w328) -> (w318:u8[])
          n135 = Reverse 1D Array(array=w319) -> (reversed array=w333:u8[])
          n136 = Reverse 1D Array(array=w317) -> (reversed array=w329:u8[])
          n137 = Reverse 1D Array(array=w318) -> (reversed array=w330:u8[])
          n138 = Reverse 1D Array(array=w312) -> (reversed array=w332:u8[])
          n139 = Reverse 1D Array(array=w322) -> (reversed array=w334:u8[])
          n140 = Reverse 1D Array(array=w311) -> (reversed array=w331:u8[])
          n141 = Reverse 1D Array(array=w323) -> (reversed array=w336:u8[])
          n142 = Reverse 1D Array(array=w325) -> (reversed array=w335:u8[])
          n143 = Type Cast(type=u16 0, x=w329) -> (*(type *) &x=w338:u16)
          n144 = Type Cast(type=w338, x=w330) -> (*(type *) &x=w339:u16)
          n145 = Type Cast(type=w339, x=w331) -> (*(type *) &x=w340:u16)
          n146 = Type Cast(type=w340, x=w332) -> (*(type *) &x=w341:u16)
          n147 = Type Cast(type=w341, x=w333) -> (*(type *) &x=w342:u16)
          n148 = Type Cast(type=w342, x=w334) -> (*(type *) &x=w343:u16)
          n149 = Type Cast(type=w343, x=w335) -> (*(type *) &x=w344:u16)
          n150 = Type Cast(type=w344, x=w336) -> (*(type *) &x=w345:u16)
          n151 = Bundle By Name(cluster=T17 {"Channel 1"=0, "Channel 2"=0, "Channel 3"=0, "Channel 4"=0, "Channel 5"=0, "Channel 6"=0, "Channel 7"=0, "Channel 8"=0} ("RC CH IN"), "Channel 1"=w338, "Channel 2"=w339, "Channel 3"=w340, "Channel 4"=w341, "Channel 5"=w342, "Channel 6"=w343, "Channel 7"=w344, "Channel 8"=w345) -> ()  [unwired: 1 out]
          n152 = call "Disable Data Stream.vi"("error in (no error)"=w307, "req_stream_id"=T15."RC_CHANNELS", "Aircraft ID"=w305) -> ("error out"=w308:errorcluster)  [unwired: 8 in]
        }
        frame 36 {
          w382 = 2 ("index")
          # "RC Channel OUT"
          n153 = String To Byte Array(string=w364) -> (unsigned byte array=w383:u8[])
          n154 = Array Subset(array=w383, index=18, length=w382) -> (w378:u8[])
          n155 = Array Subset(array=w383, index=10, length=w382) -> (w367:u8[])
          n156 = Array Subset(array=w383, index=16, length=w382) -> (w380:u8[])
          n157 = Array Subset(array=w383, index=12, length=w382) -> (w374:u8[])
          n158 = Array Subset(array=w383, index=14, length=w382) -> (w377:u8[])
          n159 = Array Subset(array=w383, index=4, length=w382) -> (w372:u8[])
          n160 = Array Subset(array=w383, index=8, length=w382) -> (w366:u8[])
          n161 = Array Subset(array=w383, index=6, length=w382) -> (w373:u8[])
          n162 = Reverse 1D Array(array=w372) -> (reversed array=w384:u8[])
          n163 = Reverse 1D Array(array=w374) -> (reversed array=w388:u8[])
          n164 = Reverse 1D Array(array=w378) -> (reversed array=w391:u8[])
          n165 = Reverse 1D Array(array=w367) -> (reversed array=w387:u8[])
          n166 = Reverse 1D Array(array=w377) -> (reversed array=w389:u8[])
          n167 = Reverse 1D Array(array=w366) -> (reversed array=w386:u8[])
          n168 = Reverse 1D Array(array=w380) -> (reversed array=w390:u8[])
          n169 = Reverse 1D Array(array=w373) -> (reversed array=w385:u8[])
          n170 = Type Cast(type=u16 0, x=w384) -> (*(type *) &x=w362:u16)
          n171 = Type Cast(type=w362, x=w385) -> (*(type *) &x=w361:u16)
          n172 = Type Cast(type=w361, x=w386) -> (*(type *) &x=w360:u16)
          n173 = Type Cast(type=w360, x=w387) -> (*(type *) &x=w359:u16)
          n174 = Type Cast(type=w359, x=w388) -> (*(type *) &x=w358:u16)
          n175 = Type Cast(type=w358, x=w389) -> (*(type *) &x=w357:u16)
          n176 = Type Cast(type=w357, x=w390) -> (*(type *) &x=w356:u16)
          n177 = Type Cast(type=w356, x=w391) -> (*(type *) &x=w355:u16)
          n178 = Bundle By Name(cluster=T17 {"Channel 1"=0, "Channel 2"=0, "Channel 3"=0, "Channel 4"=0, "Channel 5"=0, "Channel 6"=0, "Channel 7"=0, "Channel 8"=0} ("RC CH OUT"), "Channel 1"=w362, "Channel 2"=w361, "Channel 3"=w360, "Channel 4"=w359, "Channel 5"=w358, "Channel 6"=w357, "Channel 7"=w356, "Channel 8"=w355) -> ()  [unwired: 1 out]
          n179 = call "Disable Data Stream.vi"("error in (no error)"=w352, "req_stream_id"=T15."RC_CHANNELS", "Aircraft ID"=w351) -> ("error out"=w353:errorcluster)  [unwired: 8 in]
        }
        frame 39, 40, 44, 47 {
          # "Queue up mission Items in Waypoint queue including:\nMission ACK, Mission Count, Mission Item, Mission Request"
        }
        frame 77 {
          w412 = T1 {"Command ID"=0, "Command Result"=""}  # COMMAND ACK
          # "Command Acknowledge"
          n180 = String To Byte Array(string=w421) -> (unsigned byte array=w419:u8[])
          n181 = Array Subset(array=w419, length=2) -> (w423:u8[])  [unwired: 1 in]
          n182 = Array Subset(array=w419, index=2, length=1) -> (w416:u8[])
          n183 = Reverse 1D Array(array=w416) -> (reversed array=w414:u8[])
          n184 = Reverse 1D Array(array=w423) -> (reversed array=w422:u8[])
          n185 = Type Cast(type=u8 0, x=w414) -> (*(type *) &x=w413:u8)
          n186 = Type Cast(type=u16 0, x=w422) -> (*(type *) &x=w411:u16)
          n187 = case shown="4" w413 {
            tunnel: ["Command ACCEPTED and EXECUTED" "Command TEMPORARY REJECTED/DENIED" "Command PERMANENTLY DENIED" "Command UNKNOWN/UNSUPPORTED" "Command executed, but failed"] -> w399
            frame 0, Default {
            }
            frame 1 {
            }
            frame 2 {
            }
            frame 3 {
            }
            frame 4 {
            }
          }
          n188 = Unbundle By Name(w407) -> ("Status text"=w410:string)
          n189 = Concatenate Strings(w410, w399, "\n") -> ()  [unwired: 1 out]
          n190 = Bundle By Name(cluster=w412, "Command ID"=w411, "Command Result"=w399) -> (→"output cluster":T1)
          n191 = Bundle By Name(cluster=w407, "Status text"=w399) -> (w405:T5)
        }
        frame 100 {
          # "Optical Flow Data"
          n192 = call "Parse OPTICAL_FLOW.vi"("Data"=w439) -> ("Optical Flow Data"=w438:T9)  [unwired: 10 in]
          n193 = Bundle By Name(cluster=w436, "Optical Flow"=w438) -> (w435:T8)
        }
        frame 173 {
          # "Rangfinder Data"
          n194 = call "Parse RANGEFINDER.vi"("Data"=w450) -> ("Voltage"=w448:sgl, "Distance (m)"=w449:sgl)  [unwired: 9 in]
          n195 = Bundle By Name(cluster=w446, "RNGFND Distance (m)"=w449, "RNGFND Voltage"=w448) -> (w445:T8)
        }
        frame 193 {
          # "EKF Status Report"
          n196 = call "Parse EKF_STATUS_REPORT.vi"("Data"=w460) -> ("EKF Status Report"=w459:T10)  [unwired: 10 in]
          n197 = Bundle By Name(cluster=w457, "EKF Status Report"=w459) -> (w455:T8)
        }
        frame 253 {
          w469 = 100  # Max Number of Messages to Display
          # "Status Text"
          n198 = String To Byte Array(string=w481) -> (unsigned byte array=w477:u8[])
          n199 = Array Subset(array=w477, index=1, length=50) -> (w474:u8[])
          n200 = Array Subset(array=w477, length=1) -> (w479:u8[])  [unwired: 1 in]
          n201 = Byte Array To String(unsigned byte array=w474) -> (string=w472:string)
          n202 = Type Cast(type=u8 0, x=w479) -> (*(type *) &x=w471:u8)
          n203 = Unbundle By Name(w467) -> ("Status text"=w473:string)
          n204 = call "Concatenate Status Text String.vi"("Max Number of Messages to Display"=w469, "Severity"=w471, "New Status Message"=w472, "Status Text"=w473) -> ("Output"=w470:string)  [unwired: 7 in]
          n205 = Bundle By Name(cluster=w467, "Status text"=w470) -> (w466:T5)
        }
        frame Default {
          # "unknown message"
        }
      }
    }
    frame True {
      # "Timed out. nothing received\nmark coms with aircraft as bad"
      n206 = Bundle By Name(cluster=w491, "Coms with aircraft good"=FALSE) -> (w490:T11)
    }
  }
  "error in (no error) 2" <- w26
  n207 = call-poly "Aircraft Info.vi"("Aircraft ID"=w21, "Aircraft Information In"=w25) -> ("Aircraft Information Out"=w19:T11)  [unwired: 8 in, 1 out]
  n208 = feedback-in #5(w19) -> ()
  n209 = call-poly "Aircraft System Status.vi"("Aircraft ID"=w21, "System Status In"=w24) -> ("System Status Out"=w18:T5)  [unwired: 8 in, 1 out]
  n210 = feedback-in #1(w18) -> ()
  n211 = call-poly "Aircraft Extra Data.vi"("Aircraft ID"=w21, "Extra Data In"=w23) -> ("Extra Data Out"=w17:T8)  [unwired: 8 in, 1 out]
  n212 = feedback-in #4(w17) -> ()
  n213 = call-poly "Aircraft GPS.vi"("Aircraft ID"=w21, "Aircraft Att Data IN"=w22) -> ("Aircraft Att Data Out"=w16:T3)  [unwired: 8 in, 1 out]
  n214 = feedback-in #3(w16) -> ()
  n215 = call-poly "Aircraft Attitude.vi"("Aircraft ID"=w21, "Aircraft Att Data In"=w20) -> ("Aircraft Att Data Out"=w15:T2)  [unwired: 8 in, 1 out]
  n216 = feedback-in #2(w15) -> ()
